vi "poly_merge_errors_down.vi"(9 "error in 2":errorcluster, 10 "error in":errorcluster) -> (1 "error out":errorcluster)   [LabVIEW 2015]
panel:
  # "WIP"
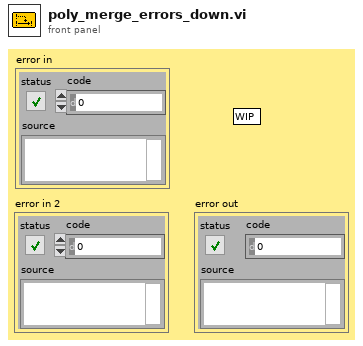
[diagram p1: front panel]
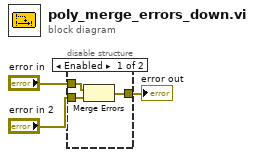
[diagram p0: block diagram]
diagram:
  n1 = disable-structure shown="Enabled" {
    disable-tunnel: "error in" -> [w6 _]
    disable-tunnel: "error in 2" -> [w5 _]
    disable-tunnel: [w4 _] -> w1
    frame Enabled {
      n2 = Merge Errors(w6, w5) -> (w4:errorcluster)
    }
    frame Disabled {
    }
  }
  "error out" <- w1
